vi "distance limit.vi"(0 "Encoder Rate":dbl, 1 "Encoder Distance":dbl, 2 "Desired Rate":dbl, 3 "Forward Limit":dbl, 5 "Reverse Limit":dbl) -> (4 "At Distance Limit":bool, 6 "Encoder Rate Out":dbl, 7 "Output Rate":dbl)   [LabVIEW 2014]
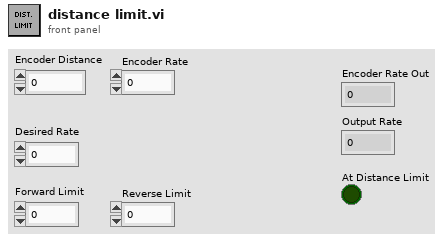
[diagram p1: front panel]
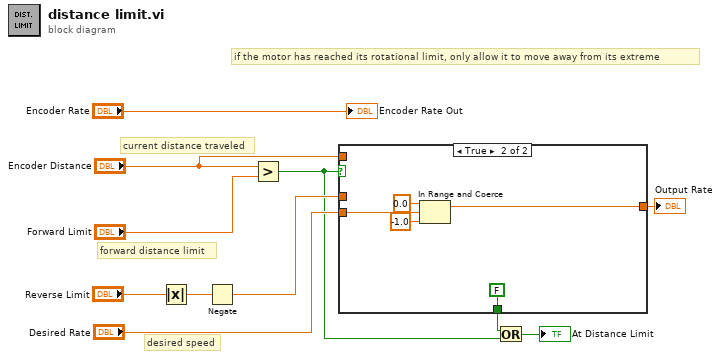
[diagram p0: block diagram]
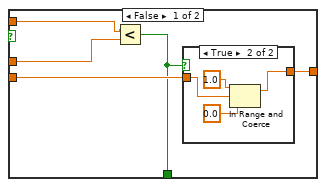
[diagram p2: hidden frame]
diagram:
  # "desired speed"
  # "forward distance limit"
  # "current distance traveled"
  # "if the motor has reached its rotational limit, only allow it to move away from its extreme"
  n1 = Absolute Value(x="Reverse Limit") -> (abs(x)=w6:dbl)
  n2 = Negate(x=w6) -> (-x=w5:dbl)
  n3 = Greater?(x="Encoder Distance", y="Forward Limit") -> (0:w3:bool)
  n4 = case shown="True" w3 {
    tunnel: "Desired Rate" -> [w15 w26]
    tunnel: "Encoder Distance" -> [w16 _]
    tunnel: [w14 w23] -> w8
    tunnel: w5 -> [w13 _]
    tunnel: [w12 FALSE] -> w4
    frame False {
      n5 = Less?(x=w16, y=w13) -> (x < y?=w12:bool)
      n6 = case shown="True" w12 {
        tunnel: w15 -> [w17 w19]
        tunnel: [w17 w18] -> w14
        frame False {
        }
        frame True {
          n7 = In Range and Coerce(upper limit=1.0, x=w19, lower limit=0.0) -> (coerced(x)=w18:dbl)  [unwired: 1 out]
        }
      }
    }
    frame True {
      n8 = In Range and Coerce(upper limit=0.0, x=w26, lower limit=-1.0) -> (coerced(x)=w23:dbl)  [unwired: 1 out]
    }
  }
  "Output Rate" <- w8
  n9 = Or(x=w4, y=w3) -> (x .or. y?=→"At Distance Limit":bool)
  "Encoder Rate Out" <- "Encoder Rate"
